vi "6 ch.vi"(0 "VISA resource name out":refnum<visa-resource-name>, 4 "Number of channels":i32, 5 "error out":errorcluster) -> (11 "output array":dbl[](array[numeric]), 12 "VISA resource name out 2":refnum<visa-resource-name>, 13 "error out 2":errorcluster, 14 "Means of 10":dbl[](array[numeric]), 15 "Means of 11":dbl[](array[numeric]), 16 "Means of 12":dbl[](array[numeric]), 17 "Means of 13":dbl[](array[numeric]), 18 "Means of 14":dbl[](array[numeric]), 19 "Means of 15":dbl[](array[numeric]))   [LabVIEW 2015]
uses:
  <instrlib>/Keithley 27XX/Public/Data/Read Multiple Direct.vi
  <instrlib>/Keithley 27XX/Keithley 27XX.lvlib
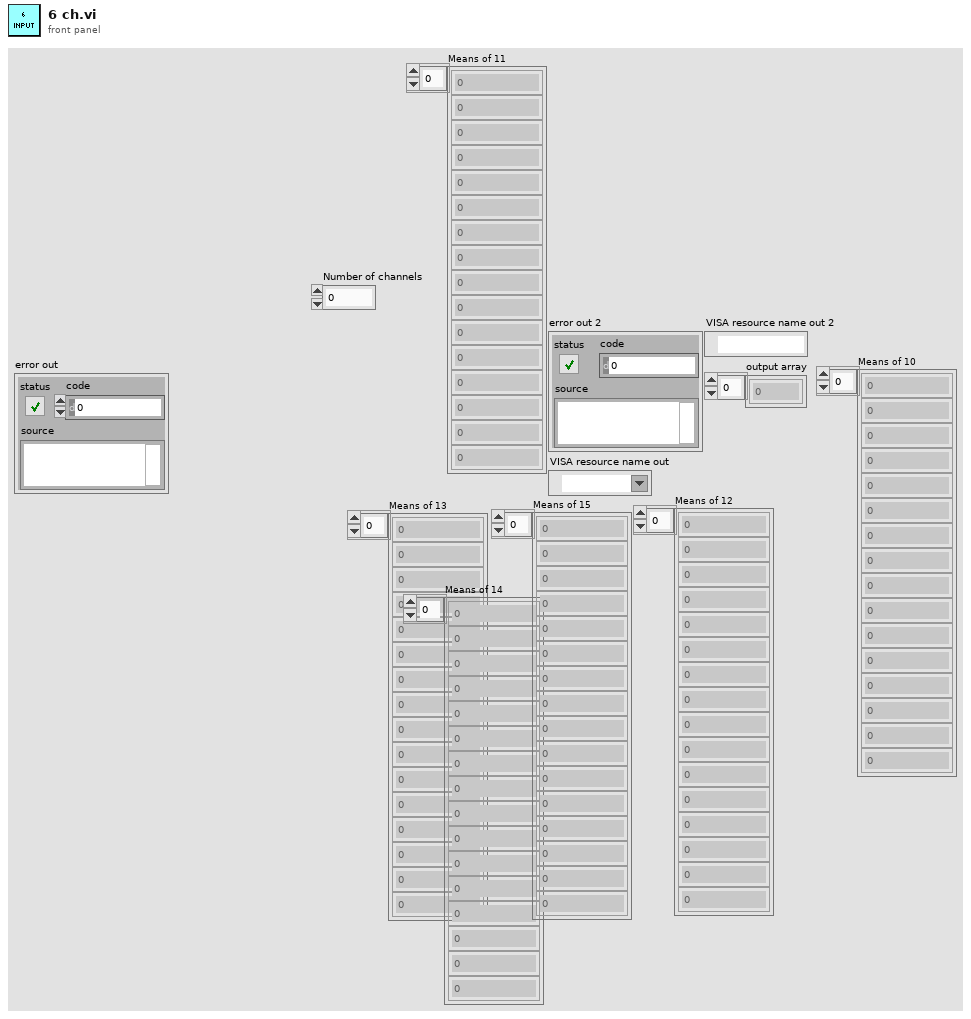
[diagram p1: front panel]
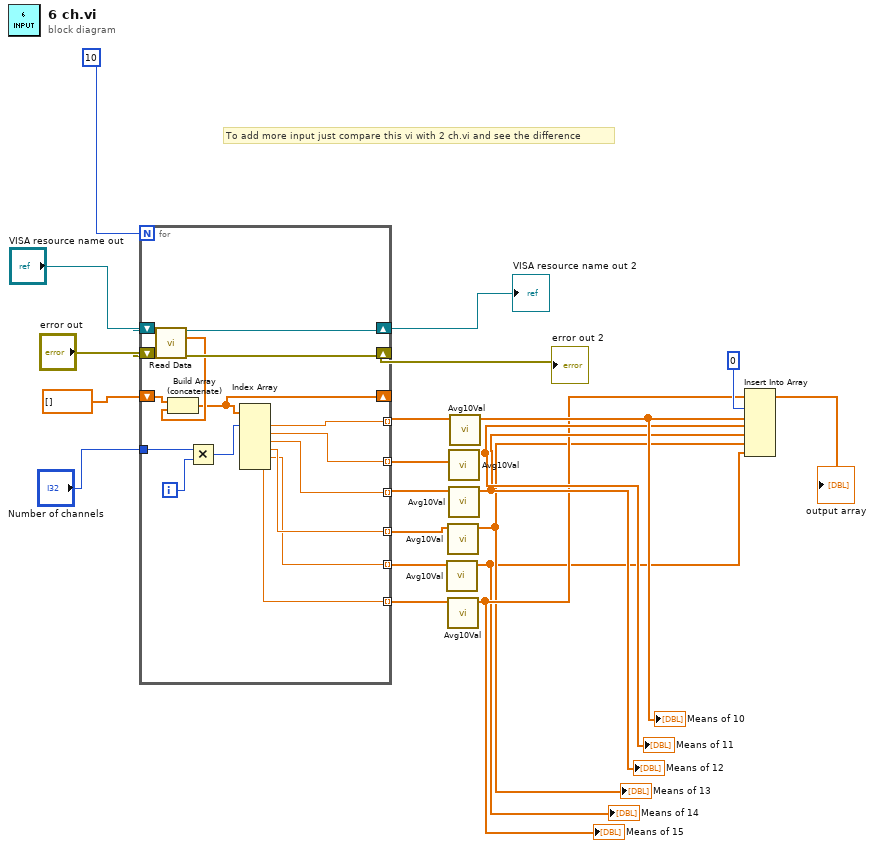
[diagram p0: block diagram]
diagram:
  # "To add more input just compare this vi with 2 ch.vi and see the difference"
  n1 = for {
    N: 10 -> [_]
    shift-right: [w36] -> w20
    shift-left: "VISA resource name out" -> [w35]
    shift-right: [w37] -> w21
    shift-left: "error out" -> [w34]
    shift-right: [w28] -> _
    shift-left: dbl[] [] -> [w33]
    tunnel: "Number of channels" -> [w30]
    tunnel: [w27] -> w16 mode=indexing
    tunnel: [w26] -> w15 mode=indexing
    tunnel: [w25] -> w10 mode=indexing
    tunnel: [w24] -> w6 mode=indexing
    tunnel: [w23] -> w5 mode=indexing
    tunnel: [w22] -> w4 mode=indexing
    i -> [w31]
    n2 = call-poly <instrlib>:"Read Data.vi"("VISA resource name"=w35, "error in (no error)"=w34) -> ("VISA resource name out"=w36:refnum<visa-resource-name>, "Measurement Data"=w32:dbl[], "error out"=w37:errorcluster)  [unwired: 8 in, 3 out]
    n3 = Build Array (concatenate)(w33, w32) -> (w28:dbl[])
    n4 = Multiply(x=w30, y=w31) -> (x*y=w29:i32)
    n5 = Index Array(array=w28, index #1=w29) -> (element #1=w27:dbl, element #2=w26:dbl, element #3=w25:dbl, element #4=w24:dbl, element #5=w23:dbl, element #6=w22:dbl)  [unwired: 5 in]
  }
  "error out 2" <- w21
  "VISA resource name out 2" <- w20
  n6 = call "Avg10Val.vi"("element"=w5) -> ("Means of 10"=w1:dbl[])  [unwired: 10 in]
  "Means of 14" <- w1
  n7 = call "Avg10Val.vi"("element"=w6) -> ("Means of 10"=w2:dbl[])  [unwired: 10 in]
  "Means of 13" <- w2
  n8 = call "Avg10Val.vi"("element"=w4) -> ("Means of 10"=w3:dbl[])  [unwired: 10 in]
  "Means of 15" <- w3
  n9 = call "Avg10Val.vi"("element"=w15) -> ("Means of 10"=w8:dbl[])  [unwired: 10 in]
  "Means of 11" <- w8
  n10 = call "Avg10Val.vi"("element"=w10) -> ("Means of 10"=w7:dbl[])  [unwired: 10 in]
  "Means of 12" <- w7
  n11 = call "Avg10Val.vi"("element"=w16) -> ("Means of 10"=w9:dbl[])  [unwired: 10 in]
  "Means of 10" <- w9
  n12 = Insert Into Array(array=w3, index=0, new element #1=w9, new element #2=w8, new element #3=w7, new element #4=w2, new element #5=w1) -> (→"output array":dbl[])
